vi "Test Delete Node From Dictionary.vi"(8 "error in (no error)":errorcluster) -> (0 "error out":errorcluster)   [LabVIEW 2017, in "Unit Tests.lvlib"]
uses:
  Unit Tests.lvlib
  source/Browser Core/Server Classes/Base Tree/Base Tree.lvclass
  source/Browser Core/Node Classes/Generic Node/Generic Node.lvclass
  source/Browser Core/Server Classes/Base Tree/Base Tree.lvclass/Base Tree.ctl
  <vilib>/addons/_JKI Toolkits/Caraya/classes/Test/Test.lvclass
  <vilib>/addons/_JKI Toolkits/Caraya/classes/Assert/Assert.lvclass
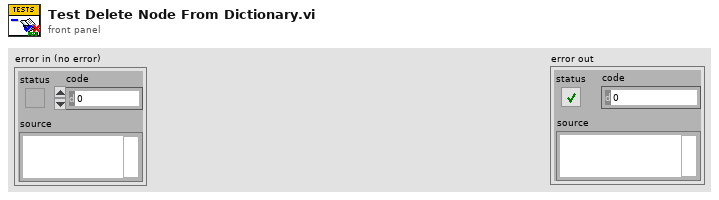
[diagram p1: front panel]
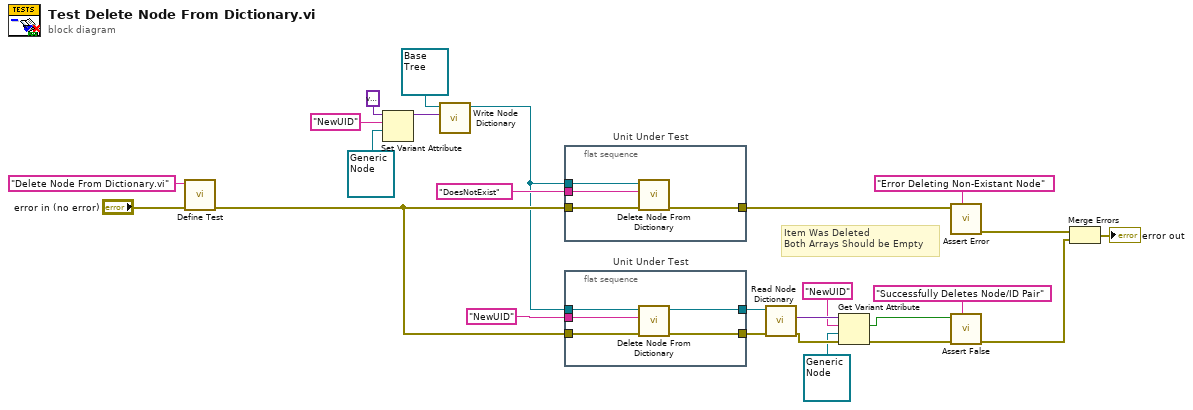
[diagram p0: block diagram]
diagram:
  # "Item Was Deleted\nBoth Arrays Should be Empty"
  n1 = call <vilib>:"Define Test.vi"("error in (no error)"="error in (no error)", "Label (VI Title)"="Delete Node From Dictionary.vi") -> ("error out"=w16:errorcluster)  [unwired: 9 in]
  n2 = Set Variant Attribute(Variant=variant ("Node Dictionary"), name="NewUID" ("UID"), value=refnum<class "Generic Node.lvclass"> refnum ("Class Node")) -> (Variant out=w10:variant)  [unwired: 1 in, 2 out]
  n3 = call "Write Node Dictionary.vi"("Node Dictionary"=w10, "Base Tree in"=refnum<class "Base Tree.lvclass"> refnum) -> ("Base Tree out"=w11:refnum<class "Base Tree.lvclass">)  [unwired: 8 in, 1 out]
  n4 = flat-sequence "Unit Under Test" {
    tunnel: w16 -> [w29]
    tunnel: "DoesNotExist" ("UID") -> [w28]
    tunnel: w11 -> [w27]
    tunnel: [w26] -> w17
    frame #0 {
      n5 = call "Delete Node From Dictionary.vi"("error in (no error)"=w29, "UID"=w28, "Base Tree in"=w27) -> ("error out"=w26:errorcluster)  [unwired: 7 in, 1 out]
    }
  }
  n6 = flat-sequence "Unit Under Test" {
    tunnel: w16 -> [w34]
    tunnel: "NewUID" ("UID") -> [w33]
    tunnel: w11 -> [w32]
    tunnel: [w31] -> w8
    tunnel: [w30] -> w7
    frame #0 {
      n7 = call "Delete Node From Dictionary.vi"("error in (no error)"=w34, "UID"=w33, "Base Tree in"=w32) -> ("error out"=w30:errorcluster, "Base Tree out"=w31:refnum<class "Base Tree.lvclass">)  [unwired: 7 in]
    }
  }
  n8 = call "Read Node Dictionary.vi"("error in (no error)"=w7, "Base Tree in"=w8) -> ("error out"=w5:errorcluster, "Node Dictionary"=w6:variant)  [unwired: 7 in, 1 out]
  n9 = Get Variant Attribute(Variant=w6, name="NewUID" ("UID"), default value (empty Variant)=refnum<class "Generic Node.lvclass"> refnum ("Class Node"), error in=w5) -> (found=w1:bool, error out=w3:errorcluster)  [unwired: 2 out]
  n10 = call <vilib>:"Assert Error.vi"("Label"="Error Deleting Non-Existant Node", "Error?"=w17) -> ("error out"=w21:errorcluster)  [unwired: 9 in]
  n11 = call <vilib>:"Assert False.vi"("Label"="Successfully Deletes Node/ID Pair", "error in (no error)"=w3, "False?"=w1) -> ("error out"=w20:errorcluster)  [unwired: 8 in]
  n12 = Merge Errors(w21, w20) -> (→"error out":errorcluster)
